vi "Update from Path.vi"(8 "error in (no error)":errorcluster, 11 "VI Reference Control in":refnum<class "VI Reference Control.lvclass">) -> (0 "error out":errorcluster, 3 "VI Reference Control out":refnum<class "VI Reference Control.lvclass">)   [LabVIEW 2016, in "VI Reference Control.lvclass"]
uses:
  VI Reference Control.lvclass
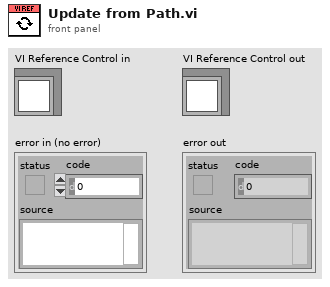
[diagram p1: front panel]
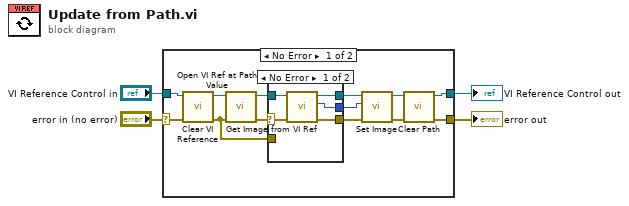
[diagram p0: block diagram]
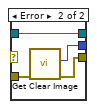
[diagram p2: hidden frame]
diagram:
  n1 = case shown="No Error" "error in (no error)" {
    selector: "error in (no error)" -> [w15 w28]
    tunnel: [w10 w28] -> w3
    tunnel: [w16 w27] -> w1
    tunnel: "VI Reference Control in" -> [w9 w27]
    frame No Error {
      n2 = call "Clear VI Reference.vi"("error in (no error)"=w15, "VI Reference Control in"=w9) -> ("error out"=w5:errorcluster, "VI Reference Control out"=w17:refnum<class "VI Reference Control.lvclass">)  [unwired: 8 in]
      n3 = call "Open VI Ref at Path Value.vi"("error in (no error)"=w5, "VI Reference Control in"=w17) -> ("error out"=w13:errorcluster, "VI Reference Control out"=w7:refnum<class "VI Reference Control.lvclass">)  [unwired: 8 in]
      n4 = case shown="No Error" w13 {
        selector: w13 -> [w22 _]
        tunnel: [w21 w24] -> w12
        tunnel: [w20 w26] -> w8
        tunnel: w7 -> [w19 w25]
        tunnel: [w18 w25] -> w6
        tunnel: w5 -> [_ w23]
        frame No Error {
          n5 = call "Get Image from VI Ref.vi"("error in (no error)"=w22, "VI Reference Control in"=w19) -> ("error out"=w21:errorcluster, "new picture"=w20:picture, "VI Reference Control out"=w18:refnum<class "VI Reference Control.lvclass">)  [unwired: 7 in]
        }
        frame Error {
          n6 = call "Get Clear Image.vi"("error in (no error)"=w23) -> ("error out"=w24:errorcluster, "Picture"=w26:picture)  [unwired: 9 in]
        }
      }
      n7 = call "Set Image.vi"("error in (no error)"=w12, "Picture"=w8, "VI Reference Control in"=w6) -> ("error out"=w11:errorcluster, "VI Reference Control out"=w14:refnum<class "VI Reference Control.lvclass">)  [unwired: 7 in]
      n8 = call "Clear Path.vi"("error in (no error)"=w11, "VI Reference Control in"=w14) -> ("error out"=w10:errorcluster, "VI Reference Control out"=w16:refnum<class "VI Reference Control.lvclass">)  [unwired: 8 in]
    }
    frame Error {
    }
  }
  "error out" <- w3
  "VI Reference Control out" <- w1
